vi "Inverse FFT PtByPt.vi"   [LabVIEW 2020, in "NI_PtbyPt.lvlib"]
doc: "Computes the inverse discrete Fourier transform (IDFT) of the set of input data points specified by <B>sample length</B>. This VI is similar to the Inverse FFT VI. Wire data to the <B>x</B> input to determine the polymorphic instance to use or manually select the instance."
uses:
  <vilib>/ptbypt/NI_PtbyPt.lvlib
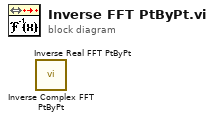
[diagram p0: block diagram]
diagram:
  n1 = call <vilib>:"Inverse Complex FFT PtByPt.vi"() -> ()  [unwired: 4 in, 2 out]
  n2 = call <vilib>:"Inverse Real FFT PtByPt.vi"() -> ()  [unwired: 4 in, 2 out]
